vi "Play_odour.vi"(6 "Odour bottles":T3(array[cluster]), 8 "error in (no error)":errorcluster, 10 "Stimulus parameters":T4, 11 "NI cluster in":T2) -> (0 "error out":errorcluster, 3 "NI cluster out":T2, 4 "AI data":waveform(dbl)[](array[waveform]))   [LabVIEW 2016]
uses:
  NI_cluster.ctl
  <vilib>/DAQmx/write.llb/DAQmx Write (Digital 1D Wfm NChan NSamp).vi
  <vilib>/DAQmx/read.llb/DAQmx Read (Analog 1D Wfm NChan NSamp).vi
  <vilib>/Waveform/DWDTOps.llb/DWDT Uncompress Digital.vi
  <vilib>/DAQmx/miscellaneous.llb/DAQmx Fill In Error Info.vi
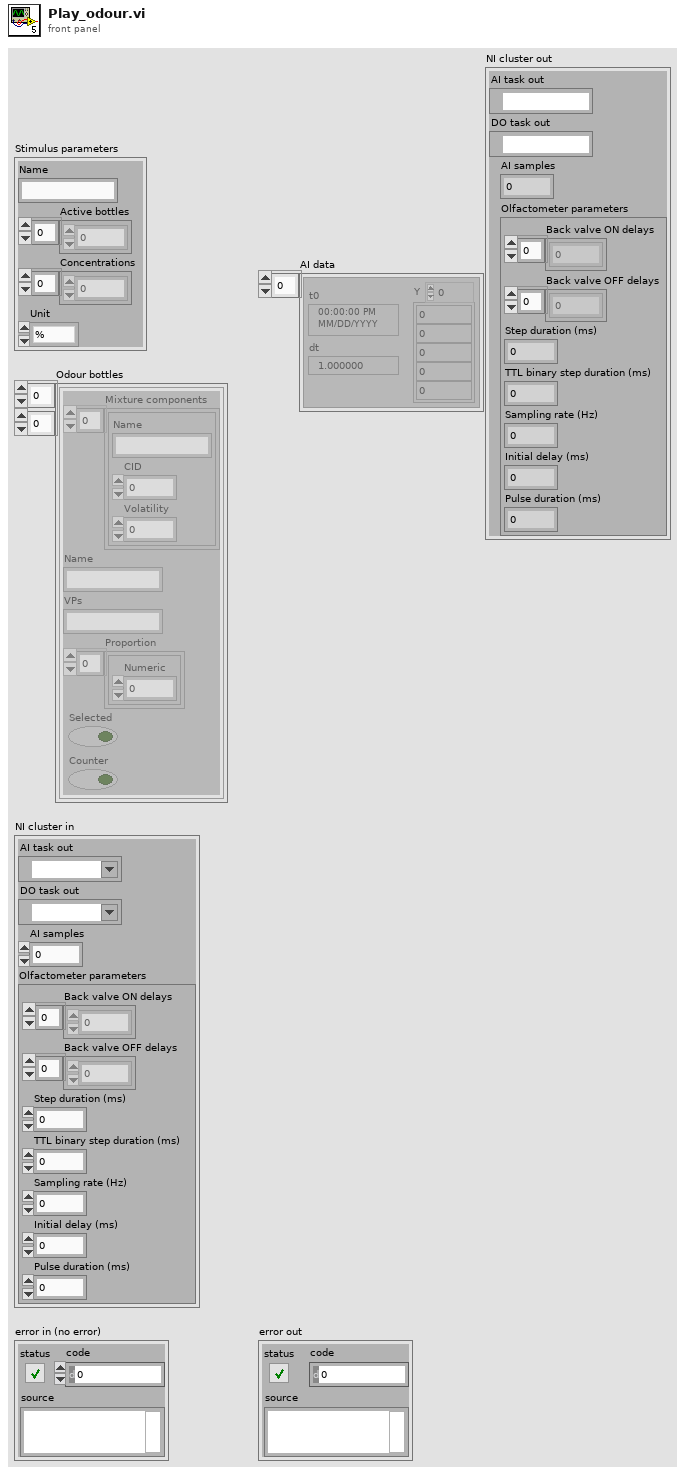
[diagram p1: front panel]
types:
  T1 = typedef "NI_cluster.ctl" = refnum<k21>
  T2 = cluster{"AI task out":refnum<k21>, "DO task out":T1, "AI samples":i32, "Olfactometer parameters":cluster{"Back valve ON delays":dbl[], "Back valve OFF delays":dbl[], "Step duration (ms)":dbl, "TTL binary step duration (ms)":dbl, "Sampling rate (Hz)":dbl, "Initial delay (ms)":dbl, "Pulse duration (ms)":dbl}}
  T3 = cluster{"Mixture components":cluster{"Name":string, "CID":i32, "Volatility":dbl}[], "Name":string, "VPs":string, "Proportion":cluster{"Numeric":dbl}[], "Selected":bool, "Counter":bool}[][]
  T4 = cluster{"Name":string, "Active bottles":i32[], "Concentrations":dbl[], "Unit":enum16{"%", "ppm"}}
  T5 = cluster{"Back valve ON delays":dbl[], "Back valve OFF delays":dbl[], "Step duration (ms)":dbl, "TTL binary step duration (ms)":dbl, "Sampling rate (Hz)":dbl, "Initial delay (ms)":dbl, "Pulse duration (ms)":dbl}
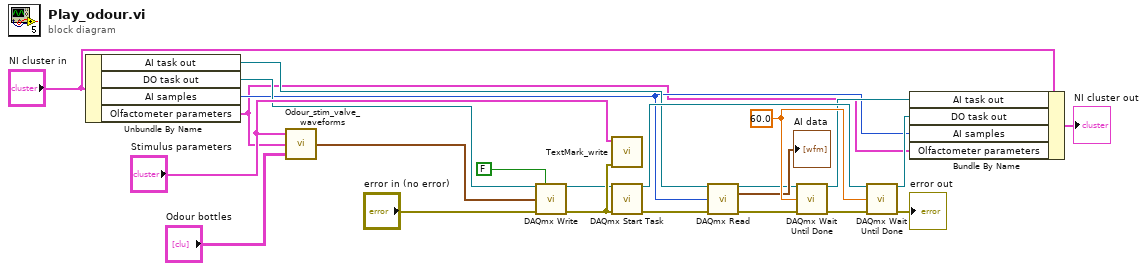
[diagram p0: block diagram]
diagram:
  w23 = 60.0 ("timeout (sec)")
  n1 = Unbundle By Name("NI cluster in") -> ("AI task out"=w10:refnum<k21>, "DO task out"=w17:T1, "AI samples"=w3:i32, "Olfactometer parameters"=w2:T5)
  n2 = call "Odour_stim_valve_waveforms.vi"("Odour bottles"="Odour bottles", "Olfactormeter parameters"=w2, "Stimulus parameters"="Stimulus parameters") -> ("waveform array"=w12:digitalwaveform[])
  n3 = call-poly <vilib>:"DAQmx Write.vi"("task/channels in"=w17, "auto start"=FALSE, "data"=w12, "error in"="error in (no error)") -> ("task out"=w13:refnum<k21>, "error out"=w19:errorcluster)  [unwired: 9 in, 1 out]
  n4 = call "TextMark_write.vi"("error in (no error)"=w19, "Stimulus parameters"="Stimulus parameters") -> ()  [unwired: 10 in]
  n5 = call <vilib>:"DAQmx Start Task.vi"("task/channels in"=w13, "error in"=w19) -> ("task out"=w14:refnum<k21>, "error out"=w15:errorcluster)  [unwired: 12 in]
  n6 = call-poly <vilib>:"DAQmx Read.vi"("task/channels in"=w10, "number of samples per channel"=w3, "error in"=w15) -> ("task out"=w8:refnum<k21>, "data"=→"AI data":waveform(dbl)[], "error out"=w16:errorcluster)  [unwired: 10 in]
  n7 = call <vilib>:"DAQmx Wait Until Done.vi"("task/channels in"=w8, "timeout (sec)"=w23, "error in"=w16) -> ("task out"=w5:refnum<k21>, "error out"=w21:errorcluster)  [unwired: 11 in]
  n8 = call <vilib>:"DAQmx Wait Until Done.vi"("task/channels in"=w14, "timeout (sec)"=w23, "error in"=w21) -> ("task out"=w4:refnum<k21>, "error out"=→"error out":errorcluster)  [unwired: 11 in]
  n9 = Bundle By Name(cluster="NI cluster in", "AI task out"=w5, "DO task out"=w4, "AI samples"=w3, "Olfactometer parameters"=w2) -> (→"NI cluster out":T2)
